vi "Dashboard Main.vi"() -> ()   [LabVIEW 2015]
uses:
  <vilib>/Utility/miscctls.llb/LVRowAndColumnTypeDef.ctl
  <vilib>/event_ctls.llb/eventvkey.ctl
  <vilib>/Rock Robotics/Network Tables/NT Write Boolean.vi
  <vilib>/Rock Robotics/WPI/Dashboard/WPI_DashboardLogging Global.vi
  <vilib>/Rock Robotics/Network Tables/NT Read Boolean.vi
  <vilib>/Utility/config.llb/Write Key (String).vi
  <vilib>/Utility/config.llb/Write Key (I32).vi
  <vilib>/Utility/config.llb/NI_LVConfig.lvlib
panel:
  out "camera num":string="Camera 1"
  out "Battery Voltage":bool
  out "timeLeft":dbl(slide) scale=0.0..150.0
  out "fps":dbl format="%#.1g"
  out "Mbps":dbl format="%#.1g"
  out "NT Connection":bool
  out "Mbps LED":bool
  in  "DB Camera Config":bool
  in  "TCP":refnum<k5>
  in  "Rec Mode":enum32{"Stop", "Record", "Playback"}(radio)
  in  "Vision":u16(ring) items=["Camera Off", "USB Camera SW", "USB Camera HW", "IP Camera"]
  out "Camera IP":string
  out "Image Message":string="Timeout in Camera Communications"
  in  "Dashboard Tab":T1(tab)
  out "Down":bool
  out "Up":bool
  out "readyToFire":bool
  out "aiming":bool
  in  "RPM setting":dbl=5400.0
  in  "Shot Mode":i32(listbox)
  in  "Defense":i32(listbox)
  in  "Autonomous Mode":i32(listbox)
  out "in range":bool
  out "back":bool
  out "forward":bool
  out "Distance":dbl
  out "Angle Off":dbl
  out "turn right":bool
  out "angleGood":bool
  out "turn left":bool
  in  "Camera Settings":T2={"Frame Rate"=30, "Compression"=30, "Size"=1} {"Frame Rate" scale=1.0..30.0; "Size" items=["640x480", "320x240", "160x120"]}
  out "Mode":T3(ring)=enum."Auto Disabled"
  out "processed image":T4(plugin-control)
  in  "rightSideSkew":dbl=0.2
  in  "leftSideSkew":dbl=1.8
  in  "compact max":dbl=1.0
  in  "compact min":dbl=0.2
  out "Shooter speed":dbl(knob) scale=0.0..6000.0
  in  "Test Slider":dbl(slide) scale=0.0..100.0 scale format="%#_3g"
  in  "On/Off":bool caption="Solenoid"
  in  "Test Name":u16(ring) items=["Select the test to run..."]
  in  "Test Tree":string(tree)
  in  "Motor":cluster{"Value":dbl, "Enable":bool} {"Value" scale=-1.0..1.0 scale format="%#_3g"}
  out "Progress":T5 {"Test Progress" scale=0.0..100.0}
  in  "Rev/Fwd":cluster{"Forward":bool, "Reverse":bool}
  in  "Test Ring":u16(ring) items=["Monochrome", "Color"]
  in  "hue max":dbl=115.0
  in  "sat max":dbl=255.0
  in  "val max":dbl=93.0
  in  "sat min":dbl=150.0
  in  "val min":dbl=9.0
  in  "hue min":dbl=90.0
  out "Cmd Status":string
  in  "Execute Command":bool
  in  "Command Params":string[][](table)
  in  "Command Selection":i32(listbox)
  in  "CheckList":i32(listbox)
  out "Tree":string(tree)
  out "Camera Image":T4(plugin-control)
  # "Range"
  # "Climber"
  # "Aim Direction"
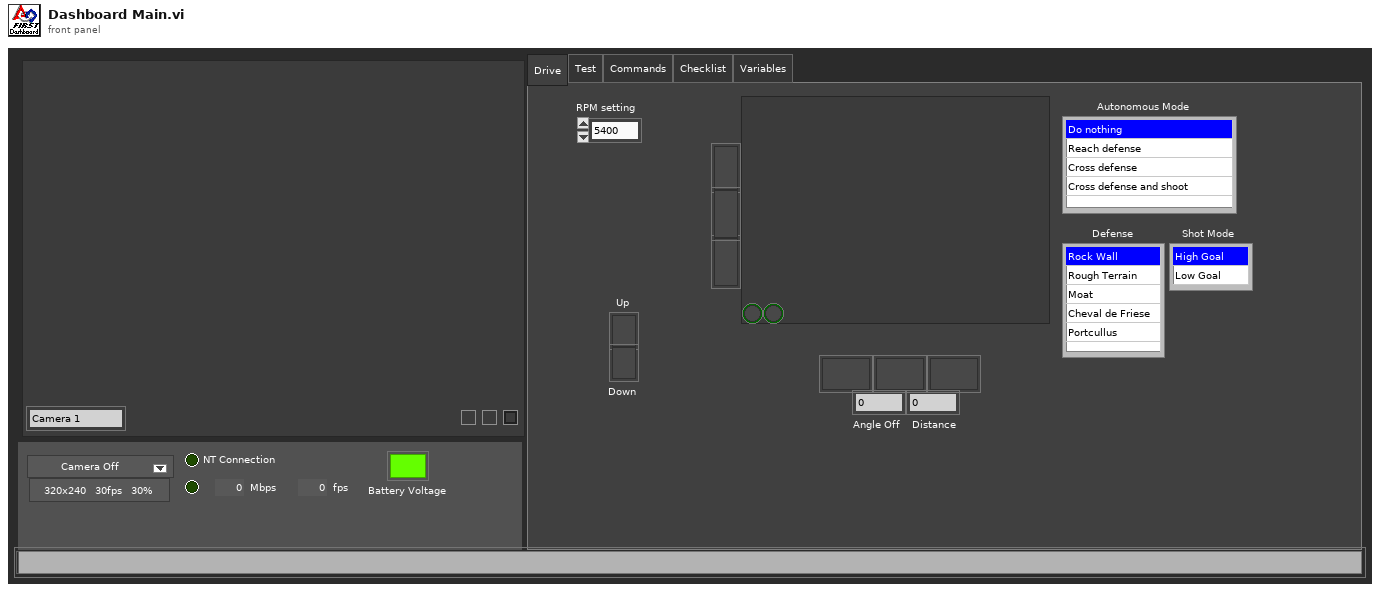
[diagram p1: front panel]
types:
  T1 = enum32{"Drive", "Test", "Commands", "Checklist", "Variables"}
  T2 = cluster{"Frame Rate":i32, "Compression":i32, "Size":u16}
  T3 = enum8{"Tele-Op Disabled", "Tele-Op Enabled", "Auto Disabled", "Auto Enabled", "Test Disabled", "Test Enabled", "Disconnected", "No Code", "E-Stop"}
  T4 = typedef "IMAQ Image.ctl" = refnum<image>
  T5 = cluster{"Test Progress":u8, "Test Progress Text":string}
  T6 = cluster{"IDs":cluster{"RPC field ID":u16, "Unique ID":u16}, "String":string}
  T7 = enum32{"Drive", "Basic", "Custom", "Test", "Checklist", "Variables"}
  T8 = typedef "Image Type" = u32
  T9 = cluster{"Error Strings":string, "Disable Counts":cluster{u16, u16}, "Rail Faults":cluster{u16, u16, u16}, "Robot IP":string, "DB Mode":u8, "Event Info":cluster{"Name":string, "Type":u8, "Number":u16, "Replay":u8}, "Camera Addr":string}
  T10 = cluster{"Storage":cluster{"Disk Free":u64, "RAM Block":u32, "RAM free":u32}, "CPU Utilization":cluster{"CPU % ISR":sgl, "CPU % Time Crit":sgl, "CPU % Timed Str":sgl, "CPU % High":sgl, "CPU % Above":sgl, "CPU % Normal":sgl, "CPU % Low":sgl}, "CAN":cluster{"% Bus Utilization":sgl, "Bus Off Cnt":u32, "TX_FIFO Full Cnt":u32, "Receive Error Cnt":u8, "Transmit Error Cnt":u8}, "HID":cluster{"HID Outputs":u32, "Rumble Low":u16, "Rumble High":u16}[]}
  T11 = cluster{"Status bits":cluster{"Test Mode":bool, "Autonomous":bool, "Enabled":bool, "Code Start":bool, "Brownout":bool, "Reserved 2":bool, "Reserved 3":bool, "E-Stop":bool}, "Code Trace":cluster{"Disabled":bool, "TeleOp":bool, "Auto":bool, "Test":bool}, "Controller Type":enum16{"unknown", "cRIO", "roboRio"}, "Code?":enum16{"unknown", "noCode", "code"}, "Battery V":dbl}
  T12 = cluster{"Control Bits":cluster{"TestMode":bool, "Autonomous":bool, "Enabled":bool, "FMS Present":bool, bool, bool, bool, "E-Stop":bool}, "Team Station ":u8, "Countdown":sgl, "Joystick Values":cluster{"Axes":dbl[], "Buttons":bool[], "POVs":i16[]}[]}
  T13 = cluster{cluster{"hue min":dbl, "hue max":dbl}, cluster{"sat min":dbl, "sat max":dbl}, cluster{"val min":dbl, "val max":dbl}}
  T14 = typedef "NI_LVConfig.lvlib/Config Data RefNum.ctl" = refnum<k1>
  T15 = cluster{"Operation":enum16{"Update", "Clear"}, "Color Box":u32}[]
  T16 = typedef "eventvkey.ctl" = enum16{"ASCII", "Enter", "Return", "Shift", "Ctrl", "Alt", "Cmd", "Opt", "Caps", "NumLock", "Clear", "Break", "Up", "Down", "Left", "Right", "Insert", "Delete", "Home", "End", "PageUp", "PageDown", "Escape", "Help", "Pause", "ScrollLock", "F1", "F2", "F3", "F4", "F5", "F6", "F7", "F8", "F9", "F10", "F11", "F12", "F13", "F14", "F15", "F16", "F17", "F18", "F19", "F20", "F21", "F22", "F23", "F24", "Play", "VolumeUp", "VolumeDown", "Mute", "Two Byte Char"}
  T17 = cluster{"Image Size":bool, "Image Type":bool, "Pixel Value":bool, "ROI Information":bool, "Zoom Factor":bool}
  T18 = enum8{"Enabled", "Disabled", "Disabled and Grayed Out"}
  T19 = cluster{"Operation":enum16{"Update", "Clear"}, "Color Box":u32}
  T20 = typedef "LVRowAndColumnTypeDef.ctl" = cluster{"Row":i32, "Column":i32}
  T21 = cluster{"Shift":bool, "Ctrl":bool, "Alt":bool, "Cmd":bool, "Opt":bool}
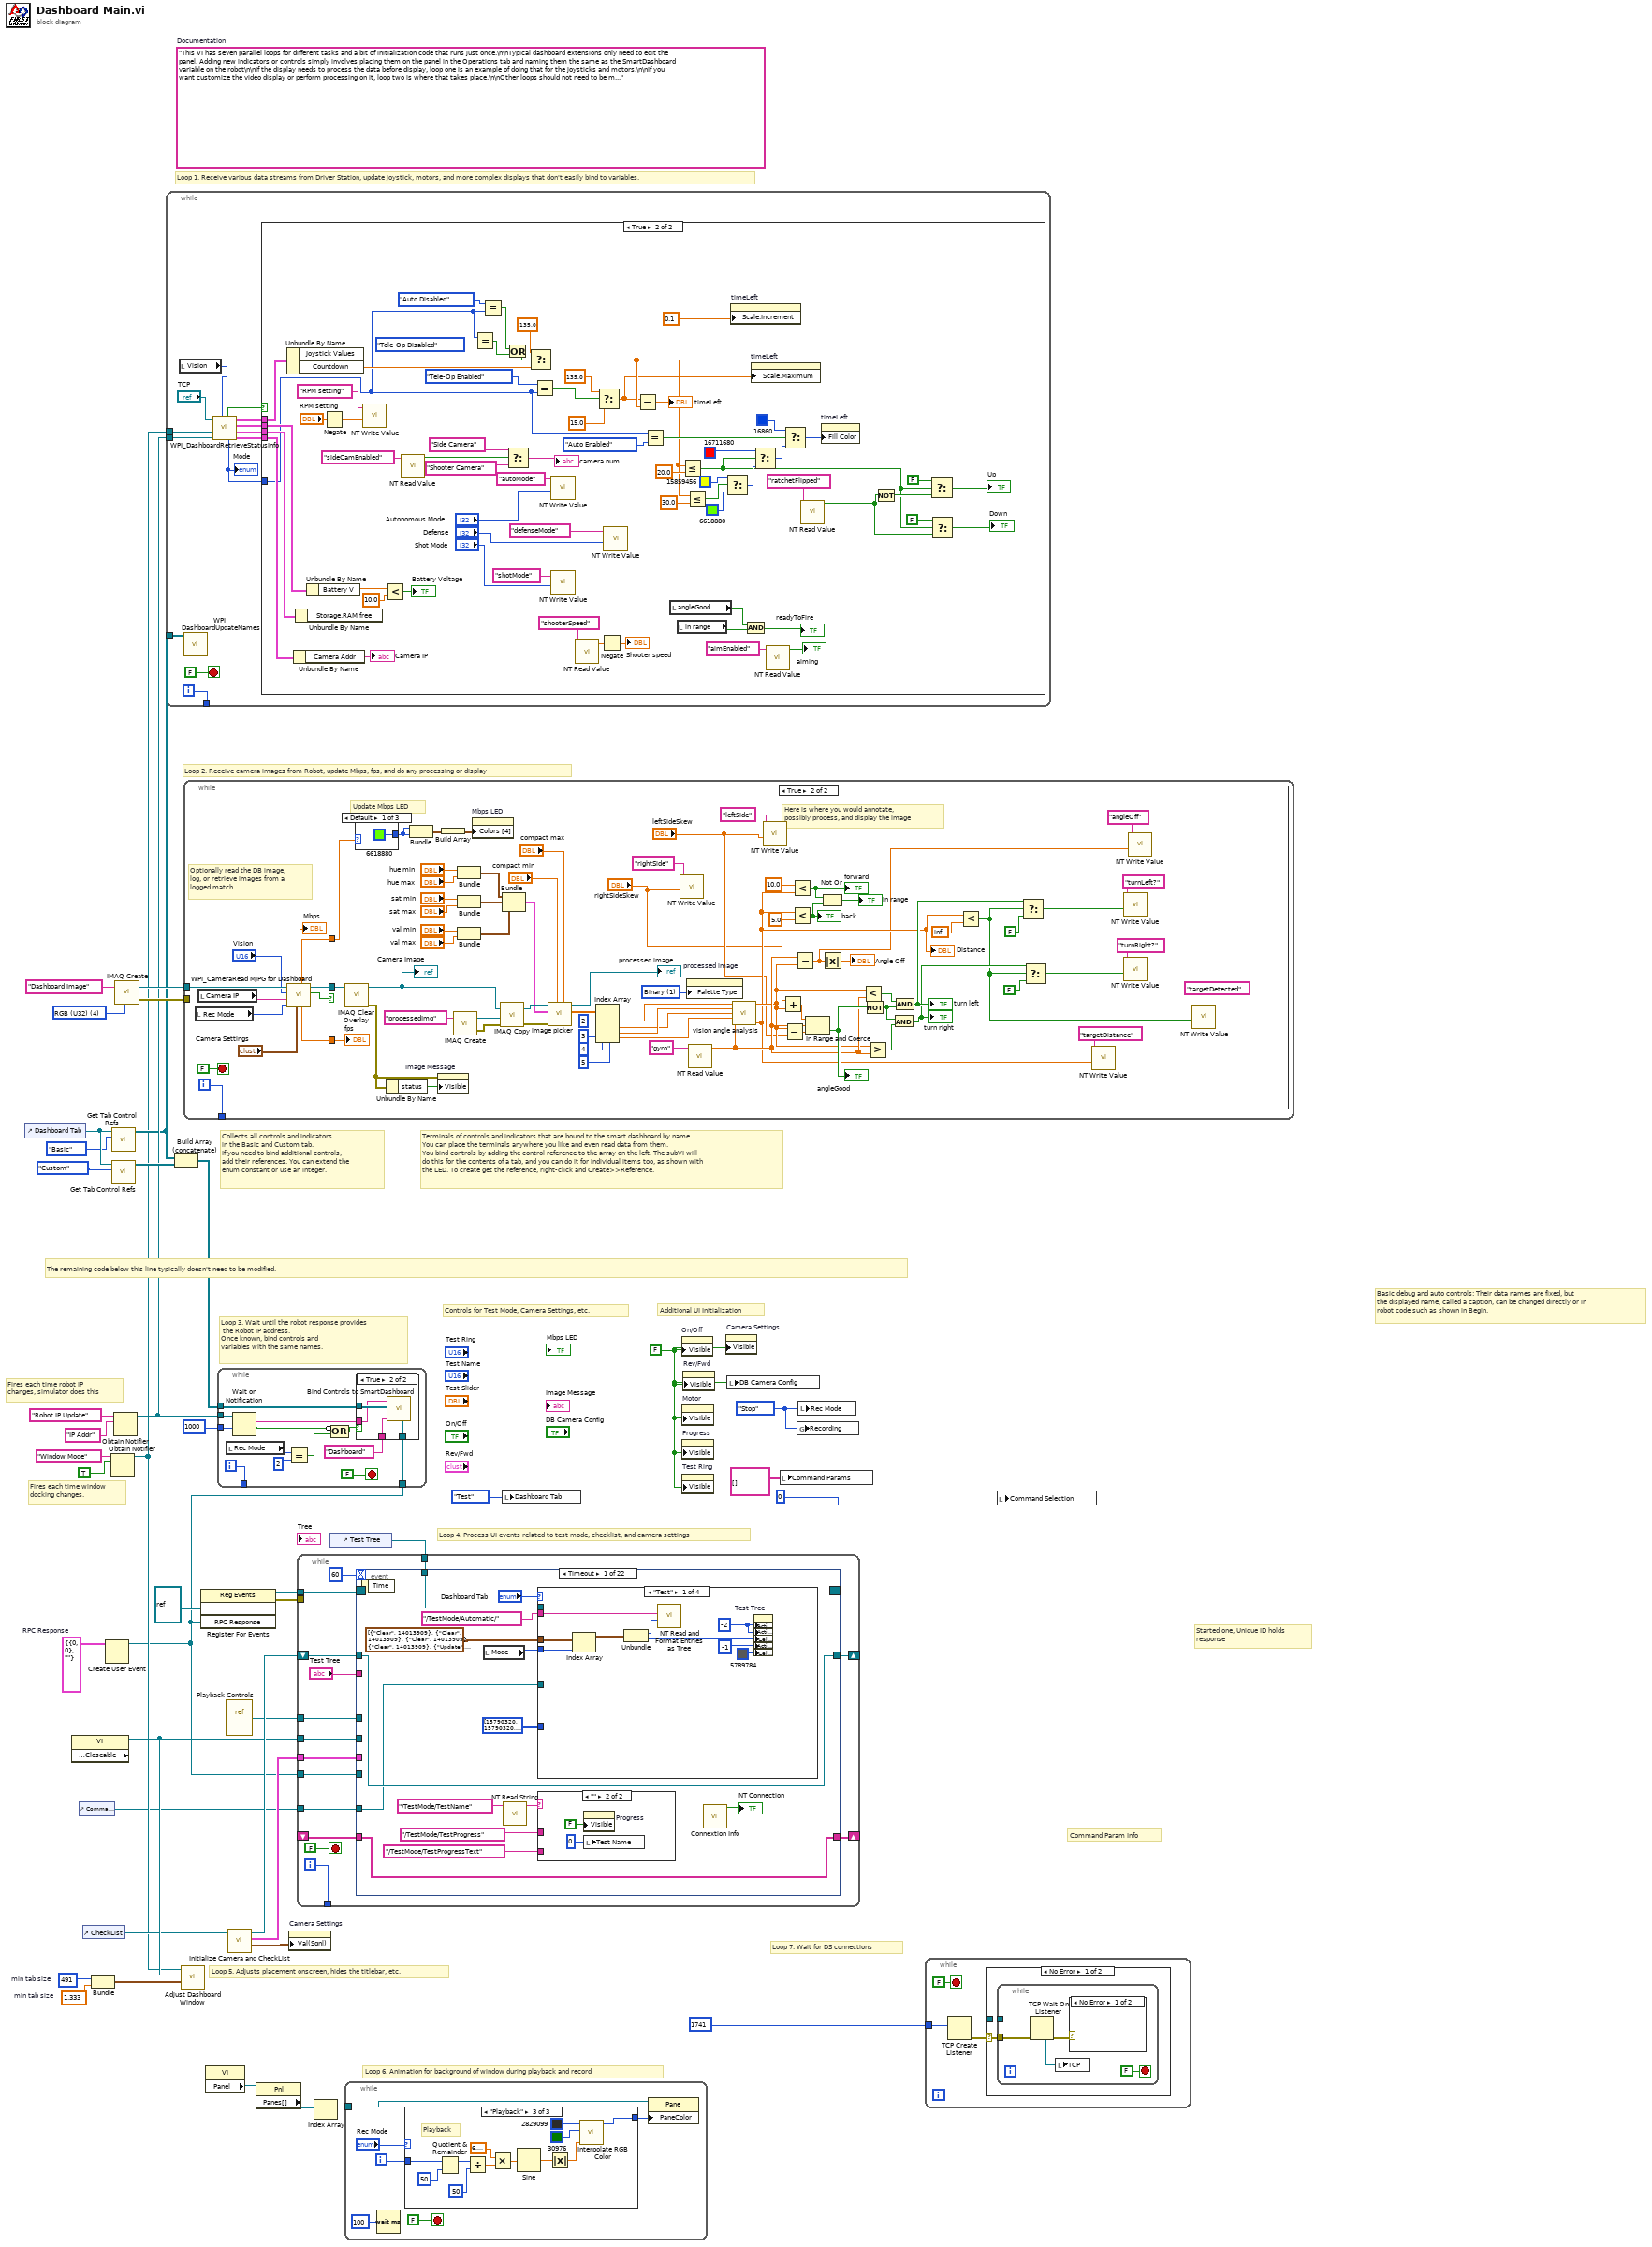
[diagram p0: block diagram]
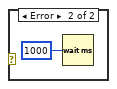
[diagram p2: hidden frame]
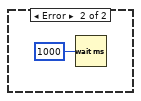
[diagram p3: hidden frame]
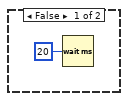
[diagram p4: hidden frame]
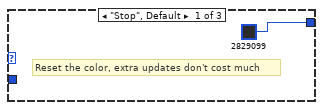
[diagram p5: hidden frame]
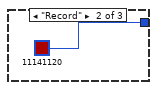
[diagram p6: hidden frame]
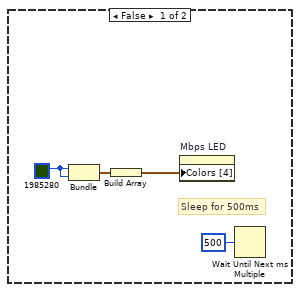
[diagram p8: hidden frame]
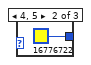
[diagram p9: hidden frame]
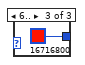
[diagram p10: hidden frame]
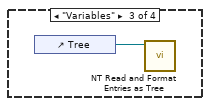
[diagram p12: hidden frame]
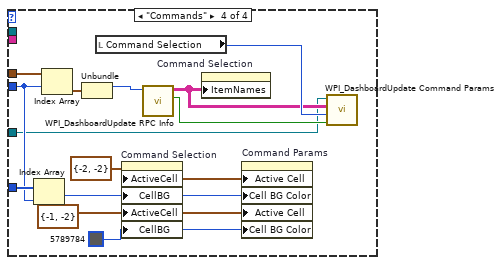
[diagram p13: hidden frame]
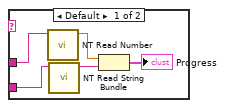
[diagram p14: hidden frame]
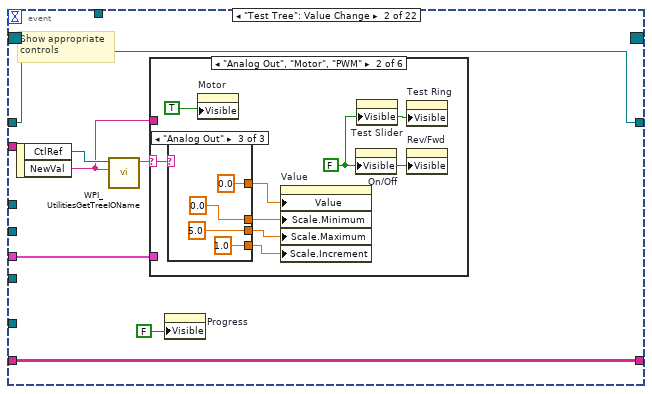
[diagram p15: hidden frame]
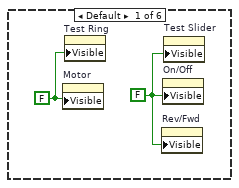
[diagram p16: hidden frame]
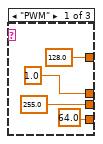
[diagram p17: hidden frame]
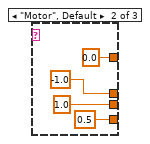
[diagram p18: hidden frame]
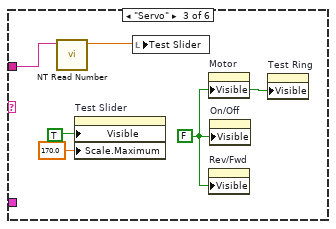
[diagram p19: hidden frame]
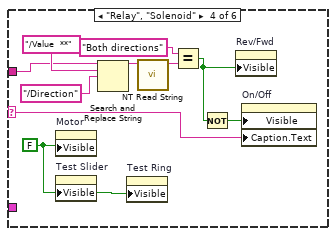
[diagram p20: hidden frame]
diagram:
  w5 = T6 {"IDs"={"RPC field ID"=0, "Unique ID"=0}, "String"=""}  # RPC Response
  w17 = 491  # min tab size
  w16 = 1.333  # min tab size
  w22 = enum32{"Stop", "Record", "Playback"}."Stop" ("Rec Mode")
  w11 = FALSE ("Visible")
  (unwired) "This VI has seven parallel loops for different tasks and a bit of initialization code that runs just once.\n\nTypical dashboard extensions only need to edit the panel. Adding new indicators or controls simply involves placing them on the panel in the Operations tab and naming them the same as the SmartDashboard variable on the robot\n\nIf the display needs to process the data before display, loop one is an example of doing that for the joysticks and motors.\n\nIf you want customize the video display or perform processing on it, loop two is where that takes place.\n\nOther loops should not need to be modified. They are pretty standard, and document the task they perform."  # Documentation
  w42 = T8 4 items=["Grayscale (U8)", "Grayscale (I16)", "Grayscale (SGL)", "Complex (CSG)", "RGB (U32)", "HSL (U32)", "RGB (U64)"] ("Image Type")
  # "Command Param Info"
  # "Started one, Unique ID holds\nresponse"
  # "Loop 7. Wait for DS connections"
  # "Basic debug and auto controls: Their data names are fixed, but\nthe displayed name, called a caption, can be changed directly or in\nrobot code such as shown in Begin."
  # "Controls for Test Mode, Camera Settings, etc."
  # "Additional UI Initialization"
  # "Loop 6. Animation for background of window during playback and record"
  # "Fires each time robot IP\nchanges, simulator does this"
  # "Fires each time window\ndocking changes."
  # "Collects all controls and indicators\nin the Basic and Custom tab.\nIf you need to bind additional controls,\nadd their references. You can extend the\nenum constant or use an integer."
  # "The remaining code below this line typically doesn't need to be modified."
  # "Loop 4. Process UI events related to test mode, checklist, and camera settings"
  # "Terminals of controls and indicators that are bound to the smart dashboard by name.\nYou can place the terminals anywhere you like and even read data from them.\nYou bind controls by adding the control reference to the array on the left. The subVI will\ndo this for the contents of a tab, and you can do it for individual items too, as shown with\nthe LED. To create get the reference, right-click and Create>>Reference."
  # "Loop 3. Wait until the robot response provides\n the Robot IP address.\nOnce known, bind controls and\nvariables with the same names."
  # "Loop 5. Adjusts placement onscreen, hides the titlebar, etc."
  # "Loop 1. Receive various data streams from Driver Station, update joystick, motors, and more complex displays that don't easily bind to variables."
  # "Loop 2. Receive camera images from Robot, update Mbps, fps, and do any processing or display"
  n1 = control-ref of="Dashboard Tab"() -> (w20:refnum<vi>)
  n2 = property class="VI" props=["Front Panel.Closeable"]() -> (reference out=w21:refnum<vi>)  [unwired: 2 in, 2 out]
  n3 = control-ref of="Command Params"() -> (w1:refnum<vi>)
  n4 = control-ref of="CheckList"() -> (w12:refnum<vi>)
  n5 = Bundle("min tab size"=w17, "min tab size"=w16) -> (w15:cluster{"min tab size":i32, "min tab size":dbl})  [unwired: 1 in]
  n6 = Create User Event(user event datatype=w5) -> (user event=w2:refnum<user-event>)  [unwired: 1 in, 1 out]
  n7 = Obtain Notifier(name (unnamed)="Window Mode", notification data type=TRUE) -> (notifier out=w8:refnum<notifier>)  [unwired: 2 in, 2 out]
  n8 = call <vilib>:"Get Tab Control Refs.vi"("Page Index"=T7."Basic" ("Dashboard Tab"), "TabControl in"=w20) -> ("ControlsOnPage"=w9:refnum<vi>[])  [unwired: 9 in]
  n9 = call <vilib>:"Get Tab Control Refs.vi"("Page Index"=T7."Custom" ("Dashboard Tab"), "TabControl in"=w20) -> ("ControlsOnPage"=w19:refnum<vi>[])  [unwired: 9 in]
  n10 = Obtain Notifier(name (unnamed)="Robot IP Update", notification data type="IP Addr" ("name (unnamed)")) -> (notifier out=w10:refnum<notifier>)  [unwired: 2 in, 2 out]
  n11 = call "IMAQ Create"("Image Name"="Dashboard Image", "Image Type"=w42) -> ("New Image"=w40:T4, "error out"=w39:errorcluster)  [unwired: 2 in, 1 out]
  n12 = while {
    tunnel: [w54] -> _
    tunnel: w10 -> [w48]
    tunnel: w9 -> [w47]
    tunnel: w8 -> [w43]
    i -> [w54]
    stop <- FALSE stop-if-true
    n13 = local read "Vision"() -> (w45:u16)
    n14 = call <vilib>:"WPI_DashboardUpdateNames.vi"("Controls on Tab"=w47) -> ()  [unwired: 11 in]
    n15 = call <vilib>:"WPI_DashboardRetrieveStatusInfo.vi"("Vision"=w45, "Binding Refnum"=w48, "Window Mode Notifier"=w43, "TCP Cnx"="TCP") -> ("Power and Errors"=w49:T9, "Robot Metrics"=w52:T10, "Status Info"=w53:T11, "Control Info"=w50:T12, "Robot Mode"=w46:T3, "Process?"=w51:bool)  [unwired: 2 in]
    "Mode" <- w46
    n16 = case shown="True" w51 {
      tunnel: w53 -> [_ w122]
      tunnel: w52 -> [_ w121]
      tunnel: w50 -> [_ w120]
      tunnel: w49 -> [_ w119]
      tunnel: w46 -> [_ w67]
      frame False {
        n17 = Wait (ms)(milliseconds to wait=u32 20) -> ()  [unwired: 1 out]
      }
      frame True {
        n18 = Unbundle By Name(w120) -> ("Countdown"=w82:sgl)  [unwired: 1 out]
        n19 = Unbundle By Name(w119) -> ("Camera Addr"=→"Camera IP":string)
        n20 = Unbundle By Name(w121) -> ()  [unwired: 1 out]
        n21 = Unbundle By Name(w122) -> ("Battery V"=w117:dbl)
        n22 = Negate(x="RPM setting") -> (-x=w94:dbl)
        n23 = call-poly <vilib>:"NT Write Value.vi"("Numeric"=w94, "Name"="RPM setting") -> ()  [unwired: 9 in, 1 out]
        n24 = Less?(x=w117, y=10.0) -> (x < y?=→"Battery Voltage":bool)
        n25 = call-poly <vilib>:"NT Read Value.vi"("Name"="sideCamEnabled") -> ("Boolean"=w111:bool)  [unwired: 9 in, 1 out]
        n26 = Equal?(x=w67, y=T3."Tele-Op Disabled") -> (x = y?=w68:bool)
        n27 = Equal?(x=T3."Auto Disabled" ("Robot Mode"), y=w67) -> (x = y?=w69:bool)
        n28 = Or(x=w69, y=w68) -> (x .or. y?=w70:bool)
        n29 = Select(t="Side Camera", s=w111, f="Shooter Camera") -> (s? t:f=→"camera num":string)
        n30 = Select(t=sgl 135.0, s=w70, f=w82) -> (s? t:f=w74:sgl)
        n31 = Equal?(x=T3."Tele-Op Enabled" ("Robot Mode"), y=w67) -> (x = y?=w76:bool)
        n32 = call-poly <vilib>:"NT Write Value.vi"("Numeric"="Autonomous Mode", "Name"="autoMode") -> ()  [unwired: 9 in, 1 out]
        n33 = call-poly <vilib>:"NT Write Value.vi"("Numeric"="Shot Mode", "Name"="shotMode") -> ()  [unwired: 9 in, 1 out]
        n34 = call-poly <vilib>:"NT Read Value.vi"("Name"="shooterSpeed") -> ("Numeric"=w105:dbl)  [unwired: 9 in, 1 out]
        n35 = Select(t=135.0, s=w76, f=15.0) -> (s? t:f=w72:dbl)
        n36 = Negate(x=w105) -> (-x=→"Shooter speed":dbl)
        n37 = call-poly <vilib>:"NT Write Value.vi"("Numeric"="Defense", "Name"="defenseMode") -> ()  [unwired: 9 in, 1 out]
        n38 = Subtract(x=w72, y=w74) -> (x-y=→"timeLeft":dbl)
        n39 = Equal?(x=w67, y=T3."Auto Enabled") -> (x = y?=w88:bool)
        n40 = local read "angleGood"() -> (w95:bool)
        n41 = local read "in range"() -> (w96:bool)
        n42 = Less Or Equal?(x=w74, y=sgl 20.0) -> (x <= y?=w59:bool)
        n43 = Less Or Equal?(x=w74, y=sgl 30.0) -> (x <= y?=w79:bool)
        n44 = Select(t=u32 15859456, s=w79, f=u32 6618880) -> (s? t:f=w80:u32)
        n45 = property on="timeLeft" class="Slide (strict)"("Scale.Increment"=0.1 ("Scale.Range:Increment")) -> ()  [unwired: 2 in, 2 out]
        n46 = And(x=w95, y=w96) -> (x .and. y?=→"readyToFire":bool)
        n47 = property on="timeLeft" class="Slide (strict)"("Scale.Maximum"=w72) -> ()  [unwired: 2 in, 2 out]
        n48 = Select(t=u32 16711680, s=w59, f=w80) -> (s? t:f=w83:u32)
        n49 = call-poly <vilib>:"NT Read Value.vi"("Name"="aimEnabled") -> ("Boolean"=→"aiming":bool)  [unwired: 9 in, 1 out]
        n50 = Select(t=u32 16860, s=w88, f=w83) -> (s? t:f=w86:u32)
        n51 = call-poly <vilib>:"NT Read Value.vi"("Name"="ratchetFlipped") -> ("Boolean"=w60:bool)  [unwired: 9 in, 1 out]
        n52 = property on="timeLeft" class="Slide (strict)"("Fill Color"=w86) -> ()  [unwired: 2 in, 2 out]
        n53 = Not(x=w60) -> (.not. x?=w61:bool)
        n54 = Select(t=FALSE, s=w59, f=w61) -> (s? t:f=→"Up":bool)
        n55 = Select(t=FALSE, s=w59, f=w60) -> (s? t:f=→"Down":bool)
      }
    }
  }
  n56 = Build Array (concatenate)(w9, w19) -> (w18:refnum<vi>[])
  n57 = call "Adjust Dashboard Window.vi"("Size Constraints"=w15, "VI"=w21, "WIn Mode"=w8) -> ()  [unwired: 9 in]
  n58 = while {
    tunnel: w40 -> [w131]
    tunnel: w39 -> [_]
    tunnel: [w132] -> _
    i -> [w132]
    stop <- FALSE stop-if-true
    # "Optionally read the DB image,\nlog, or retrieve images from a\nlogged match"
    n59 = local read "Rec Mode"() -> (w126:enum32{"Stop", "Record", "Playback"})
    n60 = local read "Camera IP"() -> (w124:string)
    n61 = call <vilib>:"WPI_CameraRead MJPG for Dashboard.vi"("Camera Settings"="Camera Settings", "Rec Mode"=w126, "Camera IP"=w124, "Camera Mode"="Vision", "Refnum in"=w131) -> ("Active"=w129:bool, "Refnum out"=w130:T4, "FPS"=w128:dbl, "Bandwidth (Mbps)"=w123:dbl)  [unwired: 3 in]
    "Mbps" <- w123
    n62 = case shown="True" w129 {
      tunnel: w130 -> [_ w204]
      tunnel: w123 -> [_ w203]
      tunnel: w128 -> [_ w202]
      frame False {
        w134 = u32 1985280 ("Color Box")
        # "Sleep for 500ms"
        n63 = Bundle("Color Box"=w134, "Color Box"=w134) -> (w136:cluster{"Color Box":u32, "Color Box":u32})  [unwired: 1 out]
        n64 = Build Array(w136) -> (w135:cluster{"Color Box":u32, "Color Box":u32}[])
        n65 = property on="Mbps LED" class="Bool (strict)"("Colors [4]"=w135) -> ()  [unwired: 2 in, 2 out]
        n66 = Wait Until Next ms Multiple(millisecond multiple=u32 500) -> ()  [unwired: 1 out]
      }
      frame True {
        w178 = u32 1 items=["Grayscale", "Binary", "Gradient", "Rainbow", "Temperature", "User Defined", "Binary 16 Bit", "Gradient 16 Bit", "Rainbow 16 Bit", "Temperature 16 Bit", "User Defined 16 Bit"] ("Palette:Palette Type")
        # "Here is where you would annotate,\npossibly process, and display the image"
        # "Update Mbps LED"
        n67 = call "IMAQ Clear Overlay"("Image"=w204) -> ("error out"=w201:errorcluster, "Image Out"=w182:T4)  [unwired: 2 in, 7 out]
        "Camera Image" <- w182
        n68 = case shown="Default" w203 {
          tunnel: [u32 6618880 ("Color Box") u32 16776722 ("Color Box") u32 16716800 ("Color Box")] -> w205
          frame Default {
          }
          frame 4, 5 {
          }
          frame 6.. {
          }
        }
        n69 = Unbundle By Name(w201) -> ("status"=w208:bool)
        n70 = Bundle("Color Box"=w205, "Color Box"=w205) -> (w207:cluster{"Color Box":u32, "Color Box":u32})  [unwired: 1 out]
        n71 = property on="Image Message" class="Str"(error in=w201, "Visible"=w208) -> ()  [unwired: 1 in, 2 out]
        n72 = Build Array(w207) -> (w206:cluster{"Color Box":u32, "Color Box":u32}[])
        n73 = call "IMAQ Create"("Image Name"="processedImg") -> ("New Image"=w181:T4, "error out"=w180:errorcluster)  [unwired: 4 in]
        n74 = Bundle("hue min"="hue min", "hue max"="hue max") -> (w175:cluster{"hue min":dbl, "hue max":dbl})  [unwired: 1 in]
        n75 = Bundle("sat min"="sat min", "sat max"="sat max") -> (w176:cluster{"sat min":dbl, "sat max":dbl})  [unwired: 1 in]
        n76 = Bundle("val min"="val min", "val max"="val max") -> (w177:cluster{"val min":dbl, "val max":dbl})  [unwired: 1 in]
        n77 = property on="Mbps LED" class="Bool (strict)"("Colors [4]"=w206) -> ()  [unwired: 2 in, 2 out]
        n78 = call "IMAQ Copy"("error in (no error)"=w180, "Image Dst"=w181, "Image Src"=w182) -> ("error out"=w184:errorcluster, "Image Dst Out"=w183:T4)  [unwired: 3 in]
        n79 = Bundle(w175, w176, w177) -> (w169:T13)  [unwired: 1 in]
        n80 = call "image picker.vi"("compactnessMax"="compact max", "compactnessMin"="compact min", "error in"=w184, "rgb constants"=w169, "Image In"=w183) -> ("report"=w167:dbl[], "Image Out"=→"processed image":T4)  [unwired: 4 in, 1 out]
        n81 = Index Array(array=w167, index #1=2 ("index"), index #2=3 ("index"), index #3=4 ("index"), index #4=5 ("index")) -> (element #1=w162:dbl, element #2=w160:dbl, element #3=w161:dbl, element #4=w159:dbl)
        n82 = call-poly <vilib>:"NT Write Value.vi"("Numeric"="rightSideSkew", "Name"="rightSide") -> ()  [unwired: 9 in, 1 out]
        n83 = property on="processed image" class="ImageControl"("Palette Type"=w178) -> ()  [unwired: 2 in, 2 out]
        n84 = call-poly <vilib>:"NT Read Value.vi"("Name"="gyro") -> ("Numeric"=w192:dbl)  [unwired: 9 in, 1 out]
        n85 = call "vision angle analysis.vi"("left_x"=w162, "right_x"=w161, "top_y"=w160, "bottom_y"=w159, "gyro_angle_deg"=w192) -> ("gyro_heading_deg"=w154:dbl, "distance"=w147:dbl)  [unwired: 9 in]
        "Distance" <- w147
        n86 = call-poly <vilib>:"NT Write Value.vi"("Numeric"="leftSideSkew", "Name"="leftSide") -> ()  [unwired: 9 in, 1 out]
        n87 = Add(x="rightSideSkew", y=w154) -> (x+y=w197:dbl)
        n88 = Subtract(x=w154, y="leftSideSkew") -> (x-y=w198:dbl)
        n89 = Less?(x=10.0, y=w147) -> (x < y?=w189:bool)
        "forward" <- w189
        n90 = Less?(x=w147, y=5.0) -> (x < y?=w188:bool)
        "back" <- w188
        n91 = Subtract(x=w192, y=w154) -> (x-y=w143:dbl)
        n92 = In Range and Coerce(upper limit=w197, x=w192, lower limit=w198) -> (In Range?=w196:bool)  [unwired: 1 out]
        "angleGood" <- w196
        n93 = Not Or(1:w188, 2:w189) -> (0:→"in range":bool)
        n94 = Absolute Value(x=w143) -> (abs(x)=→"Angle Off":dbl)
        n95 = Less?(x=w154, y=w192) -> (x < y?=w193:bool)
        n96 = Not(x=w196) -> (.not. x?=w195:bool)
        n97 = Greater?(x=w154, y=w192) -> (0:w194:bool)
        n98 = And(x=w195, y=w194) -> (x .and. y?=w150:bool)
        "turn right" <- w150
        n99 = And(x=w193, y=w195) -> (x .and. y?=w153:bool)
        "turn left" <- w153
        n100 = Less?(x=w147, y=inf) -> (x < y?=w144:bool)
        n101 = Select(t=w153, s=w144, f=FALSE) -> (s? t:f=w152:bool)
        n102 = Select(t=w150, s=w144, f=FALSE) -> (s? t:f=w148:bool)
        n103 = call-poly <vilib>:"NT Write Value.vi"("Numeric"=w147, "Name"="targetDistance") -> ()  [unwired: 9 in, 1 out]
        n104 = call-poly <vilib>:"NT Write Value.vi"("Boolean"=w152, "Name"="turnLeft?") -> ()  [unwired: 9 in, 1 out]
        n105 = call-poly <vilib>:"NT Write Value.vi"("Boolean"=w148, "Name"="turnRight?") -> ()  [unwired: 9 in, 1 out]
        n106 = call-poly <vilib>:"NT Write Value.vi"("Numeric"=w143, "Name"="angleOff") -> ()  [unwired: 9 in, 1 out]
        n107 = call-poly <vilib>:"NT Write Value.vi"("Boolean"=w144, "Name"="targetDetected") -> ()  [unwired: 9 in, 1 out]
        "fps" <- w202
      }
    }
  }
  n108 = register-events(refnum<vi> refnum, w2) -> (reference out=w26:refnum<event-registration>, error out=w25:errorcluster)  [unwired: 2 in]
  n109 = property class="VI"() -> ("Panel"=w29:refnum<vi>)  [unwired: 2 in, 2 out]
  n110 = while {
    tunnel: w18 -> [w224]
    tunnel: w10 -> [w222]
    tunnel: [w220] -> _
    tunnel: u32 1000 ("milliseconds to wait") -> [w219]
    tunnel: w2 -> [w212]
    i -> [w220]
    stop <- FALSE stop-if-true
    n111 = local read "Rec Mode"() -> (w215:enum32{"Stop", "Record", "Playback"})
    n112 = Wait on Notification(notifier=w222, timeout in ms (-1)=w219) -> (notification=w221:string, timed out?=w217:bool)  [unwired: 2 in, 2 out]
    n113 = Equal?(x=w215, y=u16 2 ("Rec Mode")) -> (x = y?=w216:bool)
    n114 = Compound Arithmetic op=OR(invert w217, w216) -> (w218:bool)
    n115 = case shown="True" w218 {
      tunnel: w224 -> [_ w228]
      tunnel: w221 -> [_ w227]
      tunnel: "Dashboard" -> [_ w226]
      tunnel: w212 -> [_ w225]
      frame False {
      }
      frame True {
        n116 = call <vilib>:"Bind Controls to SmartDashboard.vi"("RPC ref"=w225, "Client Name"=w226, "Bound Control Refs"=w228, "Server IP Address"=w227) -> ()  [unwired: 8 in]
      }
    }
  }
  n117 = vi-ref "Playback Controls.vi"() -> (w27:refnum<vi>)
  n118 = call "Initialize Camera and CheckList.vi"("ListBox in"=w12) -> ("Cluster"=w33:cluster{"value":i32, "value":i32, "index":i32}, "Array"=w34:cluster{string[]}[], "File Refnum"=w32:T14)  [unwired: 8 in]
  n119 = property class="Pnl"(reference=w29) -> ("Panes[]"=w30:refnum<vi>[])  [unwired: 1 in, 2 out]
  n120 = property on="Camera Settings" class="Clust (strict)"("Val(Sgnl)"=w33) -> ()  [unwired: 2 in, 2 out]
  n121 = Index Array(array=w30) -> (element=w28:refnum<vi>)  [unwired: 1 in]
  n122 = control-ref of="Test Tree"() -> (w31:refnum<vi>)
  n123 = while {
    tunnel: w34 -> [w240]
    shift-right: [w239] -> _
    shift-left: w32 -> [w238]
    tunnel: [w237] -> _
    tunnel: w31 -> [w236]
    tunnel: w27 -> [w235]
    tunnel: w26 -> [w234]
    tunnel: w25 -> [_]
    tunnel: w21 -> [w233]
    tunnel: w2 -> [w232]
    tunnel: w1 -> [w231]
    shift-right: [w230] -> _
    shift-left: _ -> [w229]
    i -> [w237]
    stop <- FALSE stop-if-true
    n124 = event shown="[0] Timeout" {
      selector: w234 -> [_ _ _ _ _ _ _ _ _ _ _ _ _ _ _ _ _ _ _ _ _ _]
      dyn-events: [_ _ _ _ _ _ _ _ _ _ _ _ _ _ _ _ w541 _ _ _ _ _] -> _
      timeout: u32 60 ("milliseconds to wait") -> [_ _ _ _ _ _ _ _ _ _ _ _ _ _ _ _ _ _ _ _ _ _]
      tunnel: w236 -> [w253 _ _ _ _ _ _ _ _ _ _ _ _ _ _ _ _ _ _ _ _ _]
      tunnel: "Test Tree" -> [_ _ _ _ _ _ _ _ _ _ _ w504 w513 w516 w521 w530 _ _ _ _ _ _]
      tunnel: w240 -> [_ w291 _ _ _ _ _ _ _ w466 w497 _ _ _ _ _ _ _ _ _ _ _]
      tunnel: [w250 w290 w394 w400 w412 w424 w432 w438 w451 w465 w490 w503 w511 w515 w520 w529 w543 w559 w561 w569 w580 w585] -> w239
      tunnel: w238 -> [w250 w290 w394 w400 w412 w424 w432 w438 w451 w464 w490 w503 w511 w515 w520 w529 w543 w559 w561 w569 w580 w585]
      tunnel: w235 -> [_ _ _ _ _ _ _ _ _ _ _ _ _ _ _ _ w544 _ w564 _ _ _]
      tunnel: w233 -> [_ _ _ _ _ _ _ _ _ _ _ _ _ _ _ _ w539 _ _ _ _ _]
      tunnel: w232 -> [_ _ _ _ _ _ _ _ _ _ _ _ _ _ _ _ w535 _ _ _ _ _]
      tunnel: w231 -> [w245 _ _ _ w410 _ _ _ _ _ _ _ _ _ _ _ _ _ _ _ _ _]
      tunnel: [w244 w289 w393 w399 w408 w418 w429 w437 w450 w463 w489 w502 w510 w514 w519 w528 w534 w557 w560 w565 w573 w586] -> w230
      tunnel: w229 -> [w244 w289 w393 w399 w408 _ _ w437 w450 w463 w489 w502 w510 w514 w519 w528 w534 w557 w560 w565 w573 w586]
      event Timeout {
        n125 = event-data() -> ()  [unwired: 1 in, 1 out]
        n126 = local read "Mode"() -> (w247:T3)
        n127 = call <vilib>:"NT Read String.vi"("Name"="/TestMode/TestName") -> ("String"=w256:string)  [unwired: 9 in, 1 out]
        n128 = case shown="\"Test\"" "Dashboard Tab" {
          tunnel: w253 -> [w267 _ _ _]
          tunnel: "/TestMode/Automatic/" ("Name Pattern") -> [w266 _ _ _]
          tunnel: T15 [{"Operation"=enum."Clear", "Color Box"=14013909}, {"Operation"=enum."Clear", "Color Box"=14013909}, {"Operation"=enum."Clear", "Color Box"=14013909}, {"Operation"=enum."Clear", "Color Box"=14013909}, {"Operation"=enum."Update", "Color Box"=14013909}, {"Operation"=enum."Update", "Color Box"=16777215}, {"Operation"=enum."Clear", "Color Box"=14013909}, {"Operation"=enum."Clear", "Color Box"=14013909}, {"Operation"=enum."Clear", "Color Box"=14013909}] -> [w259 _ _ w276]
          tunnel: w247 -> [w258 _ _ w275]
          tunnel: u32[] [15790320, 15790320, 15790320, 15790320, 16777215, 16777215, 15790320, 15790320, 15790320] -> [_ _ _ w281]
          tunnel: w245 -> [_ _ _ w269]
          frame "Test" {
            w265 = -2 ("Active Item:Row Number")
            n129 = Index Array(array=w259, index=w258) -> (element=w260:T19)
            n130 = Unbundle(w260) -> ("Operation"=w261:enum16{"Update", "Clear"}, "Color Box"=w262:u32)
            n131 = call <vilib>:"NT Read and Format Entries as Tree.vi"("Operation"=w261, "Name Pattern"=w266, "Tree Refnum"=w267) -> ()  [unwired: 7 in, 2 out]
            n132 = property on="Test Tree" class="Tree (strict)"("Active Item Row Number"=w265, "ActiveColNum"=w265, "CellBG"=w262, "Active Item Row Number"=-1 ("Active Item:Row Number"), "CellBG"=u32 5789784 ("Color Box")) -> ()  [unwired: 2 in, 2 out]
          }
          frame Default {
          }
          frame "Variables" {
            n133 = control-ref of="Tree"() -> (w268:refnum<vi>)
            n134 = call <vilib>:"NT Read and Format Entries as Tree.vi"("Tree Refnum"=w268) -> ()  [unwired: 9 in, 2 out]
          }
          frame "Commands" {
            w277 = u32 5789784 ("Color Box")
            w278 = T20 {"Row"=-1, "Column"=-2} ("Active Cell:Active Cell")
            w280 = T20 {"Row"=-2, "Column"=-2} ("Active Cell:Active Cell")
            n135 = Index Array(array=w281, index=w275) -> (element=w279:u32)
            n136 = Index Array(array=w276, index=w275) -> (element=w274:T19)
            n137 = Unbundle(w274) -> ("Operation"=w273:enum16{"Update", "Clear"})  [unwired: 1 out]
            n138 = local read "Command Selection"() -> (w272:i32)
            n139 = property on="Command Selection" class="MCListbox (strict)"("ActiveCell"=w280, "CellBG"=w279, "ActiveCell"=w278, "CellBG"=w277) -> ()  [unwired: 2 in, 2 out]
            n140 = call <vilib>:"WPI_DashboardUpdate RPC Info.vi"("Operation"=w273) -> ("update"=w271:bool, "commands"=w270:string[][])  [unwired: 9 in]
            n141 = property on="Command Selection" class="MCListbox (strict)"("ItemNames"=w270) -> ()  [unwired: 2 in, 2 out]
            n142 = property on="Command Params" class="Tbl (strict)"("Active Cell"=w280, "Cell BG Color"=w279, "Active Cell"=w278, "Cell BG Color"=w277) -> ()  [unwired: 2 in, 2 out]
            n143 = call <vilib>:"WPI_DashboardUpdate Command Params.vi"("Update"=w271, "NewVal"=w272, "Commands"=w270, "Param Tbl"=w269) -> ()  [unwired: 7 in, 1 out]
          }
        }
        n144 = case shown="\"\"" w256 {
          tunnel: "/TestMode/TestProgress" ("Name") -> [w283 _]
          tunnel: "/TestMode/TestProgressText" ("Name") -> [w282 _]
          frame Default {
            n145 = call <vilib>:"NT Read Number.vi"("Name"=w283) -> ("Numeric"=w284:dbl)  [unwired: 9 in, 1 out]
            n146 = call <vilib>:"NT Read String.vi"("Name"=w282) -> ("String"=w285:string)  [unwired: 9 in, 1 out]
            n147 = Bundle("Numeric"=w284, "String"=w285) -> (→"Progress":cluster{"Numeric":dbl, "String":string})  [unwired: 1 in]
          }
          frame "" {
            n148 = property on="Progress" class="Clust (strict)"("Visible"=FALSE) -> ()  [unwired: 2 in, 2 out]
            n149 = local write "Test Name"(u16 0) -> ()
          }
        }
        n150 = call <vilib>:"Connextion Info.vi"() -> ("Connected"=→"NT Connection":bool)  [unwired: 10 in, 1 out]
      }
      event "Test Tree": Value Change {
        # "Show appropriate\ncontrols"
        n151 = event-data() -> ("CtlRef"=w294:refnum<vi>, "NewVal"=w292:string)  [unwired: 1 in]
        n152 = call <vilib>:"WPI_UtilitiesGetTreeIOName.vi"("NewVal"=w292, "TreeControl in"=w294) -> ("I/O Name"=w295:string)  [unwired: 9 in]
        n153 = case shown="\"Analog Out\", \"Motor\", \"PWM\"" w295 {
          selector: w295 -> [_ w302 _ w324 w333 _]
          tunnel: w292 -> [_ _ w321 w323 _ w340]
          tunnel: w291 -> [_ _ _ _ _ w339]
          frame Default {
            w297 = FALSE ("Visible")
            w296 = FALSE ("Visible")
            n154 = property on="Motor" class="Clust (strict)"("Visible"=w296) -> ()  [unwired: 2 in, 2 out]
            n155 = property on="Test Ring" class="Ring (strict)"("Visible"=w296) -> ()  [unwired: 2 in, 2 out]
            n156 = property on="Rev/Fwd" class="Clust (strict)"("Visible"=w297) -> ()  [unwired: 2 in, 2 out]
            n157 = property on="On/Off" class="Bool (strict)"("Visible"=w297) -> ()  [unwired: 2 in, 2 out]
            n158 = property on="Test Slider" class="Slide (strict)"("Visible"=w297) -> ()  [unwired: 2 in, 2 out]
          }
          frame "Analog Out", "Motor", "PWM" {
            w303 = FALSE ("Visible")
            n159 = case shown="\"Analog Out\"" w302 {
              tunnel: [1.0 ("Value") -1.0 ("Value") 0.0 ("Value")] -> w301
              tunnel: [255.0 ("Value") 1.0 ("Value") 5.0 ("Value")] -> w300
              tunnel: [128.0 ("Value") 0.0 ("Value") 0.0 ("Value")] -> w299
              tunnel: [64.0 ("Value") 0.5 ("Value") 1.0 ("Value")] -> w298
              frame "PWM" {
              }
              frame "Motor", Default {
              }
              frame "Analog Out" {
              }
            }
            n160 = property on="Motor" class="Clust (strict)"("Visible"=TRUE) -> ()  [unwired: 2 in, 2 out]
            n161 = property on="Value" class="Slide (strict)"("Value"=w299, "Scale.Minimum"=w301, "Scale.Maximum"=w300, "Scale.Increment"=w298) -> ()  [unwired: 2 in, 2 out]
            n162 = property on="On/Off" class="Bool (strict)"("Visible"=w303) -> ()  [unwired: 2 in, 2 out]
            n163 = property on="Test Slider" class="Slide (strict)"("Visible"=w303) -> ()  [unwired: 2 in, 2 out]
            n164 = property on="Test Ring" class="Ring (strict)"("Visible"=w303) -> ()  [unwired: 2 in, 2 out]
            n165 = property on="Rev/Fwd" class="Clust (strict)"("Visible"=w303) -> ()  [unwired: 2 in, 2 out]
          }
          frame "Servo" {
            w319 = FALSE ("Visible")
            n166 = call <vilib>:"NT Read Number.vi"("Name"=w321) -> ("Numeric"=w320:dbl)  [unwired: 9 in, 1 out]
            n167 = property on="Test Slider" class="Slide (strict)"("Visible"=TRUE, "Scale.Maximum"=170.0 ("Scale.Range:Maximum")) -> ()  [unwired: 2 in, 2 out]
            n168 = local write "Test Slider"(w320) -> ()
            n169 = property on="Motor" class="Clust (strict)"("Visible"=w319) -> ()  [unwired: 2 in, 2 out]
            n170 = property on="Rev/Fwd" class="Clust (strict)"("Visible"=w319) -> ()  [unwired: 2 in, 2 out]
            n171 = property on="On/Off" class="Bool (strict)"("Visible"=w319) -> ()  [unwired: 2 in, 2 out]
            n172 = property on="Test Ring" class="Ring (strict)"("Visible"=w319) -> ()  [unwired: 2 in, 2 out]
          }
          frame "Relay", "Solenoid" {
            w322 = FALSE ("Visible")
            n173 = property on="Motor" class="Clust (strict)"("Visible"=w322) -> ()  [unwired: 2 in, 2 out]
            n174 = property on="Test Slider" class="Slide (strict)"("Visible"=w322) -> ()  [unwired: 2 in, 2 out]
            n175 = Search and Replace String(input string=w323, search string="/Value  **", replace string="/Direction") -> (result string=w329:string)  [unwired: 5 in, 3 out]
            n176 = property on="Test Ring" class="Ring (strict)"("Visible"=w322) -> ()  [unwired: 2 in, 2 out]
            n177 = call <vilib>:"NT Read String.vi"("Name"=w329) -> ("String"=w327:string)  [unwired: 9 in, 1 out]
            n178 = Equal?(x="Both directions", y=w327) -> (x = y?=w325:bool)
            n179 = Not(x=w325) -> (.not. x?=w326:bool)
            n180 = property on="Rev/Fwd" class="Clust (strict)"("Visible"=w325) -> ()  [unwired: 2 in, 2 out]
            n181 = property on="On/Off" class="Bool (strict)"("Visible"=w326, "Caption.Text"=w324) -> ()  [unwired: 2 in, 2 out]
          }
          frame "Compressor", "Digital Out" {
            w332 = FALSE ("Visible")
            # "Get direction and finish"
            n182 = property on="Motor" class="Clust (strict)"("Visible"=w332) -> ()  [unwired: 2 in, 2 out]
            n183 = property on="Test Slider" class="Slide (strict)"("Visible"=w332) -> ()  [unwired: 2 in, 2 out]
            n184 = property on="Test Ring" class="Ring (strict)"("Visible"=w332) -> ()  [unwired: 2 in, 2 out]
            n185 = property on="On/Off" class="Bool (strict)"("Visible"=TRUE, "Caption.Text"=w333) -> ()  [unwired: 2 in, 2 out]
            n186 = property on="Rev/Fwd" class="Clust (strict)"("Visible"=FALSE) -> ()  [unwired: 2 in, 2 out]
          }
          frame "Camera" {
            n187 = call <vilib>:"Get Last Path Segment.vi"("String in"=w340) -> ("String out"=w341:string)  [unwired: 10 in]
            n188 = property on="On/Off" class="Bool (strict)"("Visible"=FALSE) -> ()  [unwired: 2 in, 2 out]
            n189 = property on="Motor" class="Clust (strict)"("Visible"=FALSE) -> ()  [unwired: 2 in, 2 out]
            n190 = property on="Rev/Fwd" class="Clust (strict)"("Visible"=FALSE) -> ()  [unwired: 2 in, 2 out]
            n191 = case shown="\"White Balance  **\"" w341 {
              tunnel: w340 -> [w347 w356 w365 w374 w383 _ w389]
              tunnel: w339 -> [w345 w353 w362 w371 w380 _ _]
              frame "Size  **" {
                n192 = Index Array(array=w345) -> (element=w344:cluster{string[]})  [unwired: 1 in]
                n193 = call <vilib>:"NT Read String.vi"("Name"=w347) -> ("String"=w346:string)  [unwired: 9 in, 1 out]
                n194 = Unbundle(w344) -> (w342:string[])
                n195 = Match First String(2:w342, 3:w346) -> (0:w343:i32)  [unwired: 1 out]
                n196 = property on="Test Ring" class="Ring (strict)"("Value"=w343, "Strings []"=w342) -> ()  [unwired: 2 in, 2 out]
                n197 = property on="Test Ring" class="Ring (strict)"("Visible"=TRUE) -> ()  [unwired: 2 in, 2 out]
                n198 = property on="Test Slider" class="Slide (strict)"("Visible"=FALSE) -> ()  [unwired: 2 in, 2 out]
              }
              frame "White Balance  **" {
                n199 = Index Array(array=w353, index=1) -> (element=w354:cluster{string[]})
                n200 = call <vilib>:"NT Read String.vi"("Name"=w356) -> ("String"=w355:string)  [unwired: 9 in, 1 out]
                n201 = Unbundle(w354) -> (w351:string[])
                n202 = Match First String(2:w351, 3:w355) -> (0:w350:i32)  [unwired: 1 out]
                n203 = property on="Test Ring" class="Ring (strict)"("Value"=w350, "Strings []"=w351) -> ()  [unwired: 2 in, 2 out]
                n204 = property on="Test Ring" class="Ring (strict)"("Visible"=TRUE) -> ()  [unwired: 2 in, 2 out]
                n205 = property on="Test Slider" class="Slide (strict)"("Visible"=FALSE) -> ()  [unwired: 2 in, 2 out]
              }
              frame "Exposure  **" {
                n206 = Index Array(array=w362, index=2) -> (element=w363:cluster{string[]})
                n207 = call <vilib>:"NT Read String.vi"("Name"=w365) -> ("String"=w364:string)  [unwired: 9 in, 1 out]
                n208 = Unbundle(w363) -> (w359:string[])
                n209 = Match First String(2:w359, 3:w364) -> (0:w360:i32)  [unwired: 1 out]
                n210 = property on="Test Ring" class="Ring (strict)"("Value"=w360, "Strings []"=w359) -> ()  [unwired: 2 in, 2 out]
                n211 = property on="Test Ring" class="Ring (strict)"("Visible"=TRUE) -> ()  [unwired: 2 in, 2 out]
                n212 = property on="Test Slider" class="Slide (strict)"("Visible"=FALSE) -> ()  [unwired: 2 in, 2 out]
              }
              frame "Exposure Priority  **" {
                n213 = Index Array(array=w371, index=3) -> (element=w372:cluster{string[]})
                n214 = call <vilib>:"NT Read String.vi"("Name"=w374) -> ("String"=w373:string)  [unwired: 9 in, 1 out]
                n215 = Unbundle(w372) -> (w368:string[])
                n216 = Match First String(2:w368, 3:w373) -> (0:w369:i32)  [unwired: 1 out]
                n217 = property on="Test Ring" class="Ring (strict)"("Value"=w369, "Strings []"=w368) -> ()  [unwired: 2 in, 2 out]
                n218 = property on="Test Ring" class="Ring (strict)"("Visible"=TRUE) -> ()  [unwired: 2 in, 2 out]
                n219 = property on="Test Slider" class="Slide (strict)"("Visible"=FALSE) -> ()  [unwired: 2 in, 2 out]
              }
              frame "Color Enable  **" {
                n220 = Index Array(array=w380, index=4) -> (element=w381:cluster{string[]})
                n221 = call <vilib>:"NT Read String.vi"("Name"=w383) -> ("String"=w382:string)  [unwired: 9 in, 1 out]
                n222 = Unbundle(w381) -> (w377:string[])
                n223 = Match First String(2:w377, 3:w382) -> (0:w378:i32)  [unwired: 1 out]
                n224 = property on="Test Ring" class="Ring (strict)"("Value"=w378, "Strings []"=w377) -> ()  [unwired: 2 in, 2 out]
                n225 = property on="Test Ring" class="Ring (strict)"("Visible"=TRUE) -> ()  [unwired: 2 in, 2 out]
                n226 = property on="Test Slider" class="Slide (strict)"("Visible"=FALSE) -> ()  [unwired: 2 in, 2 out]
              }
              frame Default {
                n227 = property on="Test Ring" class="Ring (strict)"("Visible"=FALSE) -> ()  [unwired: 2 in, 2 out]
                n228 = property on="Test Slider" class="Slide (strict)"("Visible"=FALSE) -> ()  [unwired: 2 in, 2 out]
              }
              frame "Brightness  **", "Color Level  **", "Compression  **", "FPS  **", "Sharpness  **" {
                n229 = call <vilib>:"NT Read Number.vi"("Name"=w389) -> ("Numeric"=w388:dbl)  [unwired: 9 in, 1 out]
                n230 = local write "Test Slider"(w388) -> ()
                n231 = property on="Test Slider" class="Slide (strict)"("Visible"=TRUE, "Scale.Maximum"=100.0 ("Scale.Range:Maximum")) -> ()  [unwired: 2 in, 2 out]
                n232 = property on="Test Ring" class="Ring (strict)"("Visible"=FALSE) -> ()  [unwired: 2 in, 2 out]
              }
            }
          }
        }
        n233 = property on="Progress" class="Clust (strict)"("Visible"=FALSE) -> ()  [unwired: 2 in, 2 out]
      }
      event "Test Name": Mouse Enter {
        # "Populate the ring with the list of tests"
        n234 = event-data() -> ()  [unwired: 1 in, 1 out]
        n235 = call <vilib>:"NT Read String Array.vi"("Name"="/TestMode/TestList") -> ("String Array"=w398:string[])  [unwired: 9 in, 1 out]
        n236 = Build Array (concatenate)("Select the test to run...", w398) -> (w397:string[])
        n237 = property on="Test Name" class="Ring (strict)"("Strings []"=w397) -> ()  [unwired: 2 in, 2 out]
      }
      event "Test Name": Value Change {
        w401 = FALSE ("Visible")
        # "Tell the robot the test name to run"
        n238 = event-data() -> ("NewVal"=w405:u16)  [unwired: 1 in]
        n239 = property on="Test Name" class="Ring (strict)"() -> ("Strings []"=w406:string[])  [unwired: 2 in, 2 out]
        n240 = local write "Progress"(T5 {"Test Progress"=0, "Test Progress Text"=""} ("Progress")) -> ()
        n241 = Index Array(array=w406, index=w405) -> (element=w404:string)
        n242 = call <vilib>:"NT Write String.vi"("String"=w404, "Name"="/TestMode/TestName") -> ()  [unwired: 9 in, 1 out]
        n243 = property on="Progress" class="Clust (strict)"("Visible"=TRUE) -> ()  [unwired: 2 in, 2 out]
        n244 = property on="Motor" class="Clust (strict)"("Visible"=w401) -> ()  [unwired: 2 in, 2 out]
        n245 = property on="Test Slider" class="Slide (strict)"("Visible"=w401) -> ()  [unwired: 2 in, 2 out]
        n246 = property on="On/Off" class="Bool (strict)"("Visible"=w401) -> ()  [unwired: 2 in, 2 out]
        n247 = property on="Rev/Fwd" class="Clust (strict)"("Visible"=w401) -> ()  [unwired: 2 in, 2 out]
        n248 = property on="Test Ring" class="Ring (strict)"("Visible"=w401) -> ()  [unwired: 2 in, 2 out]
      }
      event "Command Selection": Value Change {
        # "Get the params and show in table"
        n249 = event-data() -> ("NewVal"=w411:i32)  [unwired: 1 in]
        n250 = property on="Command Selection" class="MCListbox (strict)"() -> ("ItemNames"=w409:string[][])  [unwired: 2 in, 2 out]
        n251 = call <vilib>:"WPI_DashboardUpdate Command Params.vi"("NewVal"=w411, "Commands"=w409, "Param Tbl"=w410) -> ()  [unwired: 8 in, 1 out]
      }
      event "Execute Command": Value Change {
        # "Started one, Unique ID holds\nresponse"
        n252 = event-data() -> ()  [unwired: 1 in, 1 out]
        n253 = property on="Command Selection" class="MCListbox (strict)"() -> ("ItemNames"=w423:string[][])  [unwired: 2 in, 2 out]
        n254 = Index Array(array=w423, index (row)="Command Selection", index (col)=0) -> (element=w421:string)
        n255 = call <vilib>:"Invoke Commands.vi"("Command Params"="Command Params", "Function Name"=w421) -> ("Params"=w417:u8, "Started"=w416:bool)  [unwired: 7 in, 1 out]
        n256 = Array Subset(array="Command Params", length (row)=w417) -> (w418:string[][])  [unwired: 3 in]
        n257 = Select(t="Executing" ("Cmd Status"), s=w416, f="" ("Cmd Status")) -> (s? t:f=→"Cmd Status":string)
      }
      event "Command Selection": Double Click {
        n258 = event-data() -> ("Row"=w433:i32)  [unwired: 1 in]
        n259 = property on="Command Selection" class="MCListbox (strict)"() -> ("ItemNames"=w436:string[][])  [unwired: 2 in, 2 out]
        n260 = local read "Command Params"() -> (w431:string[][])
        n261 = Index Array(array=w436, index (row)=w433, index (col)=0) -> (element=w434:string)
        n262 = call <vilib>:"Invoke Commands.vi"("Command Params"=w431, "Function Name"=w434) -> ("Params"=w430:u8, "Started"=w425:bool)  [unwired: 7 in, 1 out]
        n263 = Array Subset(array=w431, length (row)=w430) -> (w429:string[][])  [unwired: 3 in]
        n264 = Select(t="Executing" ("Cmd Status"), s=w425, f="" ("Cmd Status")) -> (s? t:f=w426:string)
        n265 = local write "Cmd Status"(w426) -> ()
      }
      event "CheckList": Double Click {
        # "Shift clears all"
        # "Update symbols on the listbox"
        n266 = event-data() -> ("PlatMods.Shift"=w439:bool, "Row"=w441:i32)  [unwired: 1 in]
        n267 = case shown="True" w439 {
          tunnel: w441 -> [w445 _]
          tunnel: 1 -> [w444 _]
          frame False {
            n268 = property on="CheckList" class="LstBox (strict)"() -> ("Item Symbols"=w443:i32[])  [unwired: 2 in, 2 out]
            n269 = Replace Array Subset(array=w443, new element=w444, index=w445) -> (w442:i32[])
            n270 = property on="CheckList" class="LstBox (strict)"("Item Symbols"=w442) -> ()  [unwired: 2 in, 2 out]
          }
          frame True {
            w446 = 0 ("Top Row")
            n271 = property on="CheckList" class="LstBox (strict)"() -> ("Number of Rows"=w448:u32)  [unwired: 2 in, 2 out]
            n272 = Initialize Array(0, w448) -> (w447:i32[])
            n273 = property on="CheckList" class="LstBox (strict)"("Top Row"=w446, "Value"=w446, "Item Symbols"=w447) -> ()  [unwired: 2 in, 2 out]
          }
        }
      }
      event "CheckList": Key Down {
        # "Update symbols on the listbox\nLeft and right keys check and uncheck"
        n274 = event-data() -> ("VKey"=w453:T16)  [unwired: 1 in]
        n275 = case shown="\"Left\", \"Right\"" w453 {
          selector: w453 -> [w458 _]
          tunnel: eventvkey."Left" ("VKey") -> [w456 _]
          frame "Left", "Right" {
            n276 = Equal?(x=w456, y=w458) -> (x = y?=w457:bool)
            n277 = Select(t=0, s=w457, f=1) -> (s? t:f=w459:i32)
            n278 = property on="CheckList" class="LstBox (strict)"() -> ("Item Symbols"=w462:i32[])  [unwired: 2 in, 2 out]
            n279 = Replace Array Subset(array=w462, new element=w459, index="CheckList") -> (w461:i32[])
            n280 = property on="CheckList" class="LstBox (strict)"("Item Symbols"=w461) -> ()  [unwired: 2 in, 2 out]
          }
          frame Default {
          }
        }
      }
      event "DB Camera Config": Value Change {
        # "Show or hide the cluster of controls, store in ini file"
        n281 = event-data() -> ("NewVal"=w467:bool)  [unwired: 1 in]
        n282 = case shown="False" w467 {
          tunnel: w466 -> [w476 _]
          tunnel: [w469 w487] -> w465
          tunnel: w464 -> [w468 w487]
          frame False {
            w483 = "Camera"
            w486 = FALSE ("Visible")
            n283 = local read "Camera Settings"() -> (w475:T2)
            n284 = Index Array(array=w476) -> (element=w479:cluster{string[]})  [unwired: 1 in]
            n285 = Unbundle(w475) -> ("Frame Rate"=w474:i32, "Compression"=w473:i32, "Size"=w477:u16)
            n286 = Unbundle(w479) -> (w478:string[])
            n287 = Index Array(array=w478, index=w477) -> (element=w472:string)
            n288 = call-poly <vilib>:"Write Key.vi"("section"=w483, "value"=w472, "key"="Size", "refnum"=w468) -> ("refnum out"=w485:T14)  [unwired: 2 in, 5 out]
            n289 = call-poly <vilib>:"Write Key.vi"("section"=w483, "value"=w474, "key"="FrameRate", "refnum"=w485) -> ("refnum out"=w484:T14)  [unwired: 1 in, 6 out]
            n290 = property on="Camera Settings" class="Clust (strict)"("Visible"=w486) -> ()  [unwired: 2 in, 2 out]
            n291 = local write "DB Camera Config"(w486) -> ()
            n292 = call-poly <vilib>:"Write Key.vi"("section"=w483, "value"=w473, "key"="Compression", "refnum"=w484) -> ("refnum out"=w470:T14)  [unwired: 1 in, 6 out]
            n293 = call <vilib>:"Close Config Data.vi"("refnum"=w470) -> ("file path"=w471:path)  [unwired: 2 in, 8 out]
            n294 = call <vilib>:"Open Config Data.vi"("configuration file path"=w471) -> ("refnum"=w469:T14)  [unwired: 8 in, 2 out]
          }
          frame True {
            n295 = property on="Camera Settings" class="Clust (strict)"("Visible"=TRUE) -> ()  [unwired: 2 in, 2 out]
          }
        }
      }
      event "Camera Settings": Value Change {
        # "Update summary string when any elements of DB camera change"
        n296 = event-data() -> ("NewVal"=w501:T2)  [unwired: 1 in]
        n297 = Index Array(array=w497) -> (element=w496:cluster{string[]})  [unwired: 1 in]
        n298 = Unbundle(w501) -> ("Frame Rate"=w492:i32, "Compression"=w491:i32, "Size"=w494:u16)
        n299 = Unbundle(w496) -> (w495:string[])
        n300 = Index Array(array=w495, index=w494) -> (element=w493:string)
        n301 = Format Into String(format string="%s   %dfps   %d%%", w493, w492, w491) -> (resulting string=w498:string)  [unwired: 2 in, 1 out]
        n302 = Build Array(w498) -> (w499:string[])
        n303 = property on="DB Camera Config" class="Bool (strict)"("Strings [4]"=w499) -> ()  [unwired: 2 in, 2 out]
      }
      event "Motor.Enable": Value Change {
        # "When the test mode otor enable helper is set, update that\ntree row item's value"
        n304 = event-data() -> ("NewVal"=w508:bool)  [unwired: 1 in]
        n305 = Unbundle("Motor") -> ("Value"=w507:dbl)  [unwired: 1 out]
        n306 = Select(t=w507, s=w508, f=0.0) -> (s? t:f=w505:dbl)
        n307 = call <vilib>:"NT Write Number.vi"("Numeric"=w505, "Name"=w504) -> ()  [unwired: 9 in, 1 out]
      }
      event "Test Slider": Value Change {
        # "When the test mode slider helper is set, update that\ntree row item's value"
        n308 = event-data() -> ("NewVal"=w512:dbl)  [unwired: 1 in]
        n309 = call <vilib>:"NT Write Number.vi"("Numeric"=w512, "Name"=w513) -> ()  [unwired: 9 in, 1 out]
      }
      event "On/Off": Value Change {
        # "When the test mode on/off helper value is set, update that\ntree row item's value"
        n310 = event-data() -> ("NewVal"=w518:bool)  [unwired: 1 in]
        n311 = Boolean To (0,1)(Boolean=w518) -> (0, 1=w517:i16)
        n312 = call <vilib>:"NT Write Number.vi"("Numeric"=w517, "Name"=w516) -> ()  [unwired: 9 in, 1 out]
      }
      event "Rev/Fwd": Value Change {
        # "When the test mode helper value for relays is set, update that\ntree row item's value"
        n313 = event-data() -> ("NewVal.Forward"=w527:bool, "NewVal.Reverse"=w526:bool)  [unwired: 1 in]
        n314 = Boolean To (0,1)(Boolean=w527) -> (0, 1=w523:i16)
        n315 = Boolean To (0,1)(Boolean=w526) -> (0, 1=w525:i16)
        n316 = Negate(x=w525) -> (-x=w524:i16)
        n317 = Add(x=w523, y=w524) -> (x+y=w522:i16)
        n318 = call <vilib>:"NT Write Number.vi"("Numeric"=w522, "Name"=w521) -> ()  [unwired: 9 in, 1 out]
      }
      event "Test Ring": Value Change {
        # "When a test mode helper value is selected from the ring,\nset the tree item's variable to the string value"
        n319 = event-data() -> ("NewVal"=w532:u16)  [unwired: 1 in]
        n320 = property on="Test Ring" class="Ring (strict)"() -> ("Strings []"=w533:string[])  [unwired: 2 in, 2 out]
        n321 = Index Array(array=w533, index=w532) -> (element=w531:string)
        n322 = call <vilib>:"NT Write String.vi"("String"=w531, "Name"=w530) -> ()  [unwired: 9 in, 1 out]
      }
      event "Rec Mode": Value Change {
        # "Update globals for recording mode and path to read log from.\nClear when logging and let NetworkTables set path for vision to\nuse."
        n323 = event-data() -> ("NewVal"=w545:enum32{"Stop", "Record", "Playback"})  [unwired: 1 in]
        n324 = global write "WPI_DashboardLogging Global.vi" "Logging Filename"(path "") -> ()
        n325 = global write "WPI_DashboardLogging Global.vi" "Recording"(w545) -> ()
        n326 = case shown="\"Playback\"" w545 {
          tunnel: w544 -> [_ w547 w556]
          tunnel: [_ _ w555] -> w541
          tunnel: [_ _ w554] -> _
          tunnel: w539 -> [_ _ w552]
          tunnel: cluster{i32, i32} {-250, 170} -> [_ _ w551]
          tunnel: [_ _ T17 {"Image Size"=TRUE, "Image Type"=TRUE, "Pixel Value"=TRUE, "ROI Information"=TRUE, "Zoom Factor"=FALSE} ("Image Information Shown:All Elements")] -> w537
          tunnel: [_ _ TRUE ("Zoom Factor")] -> w536
          tunnel: w535 -> [_ _ w548]
          frame Default {
          }
          frame "Stop", "Record" {
            # "Place Window too"
            n327 = invoke class="VI" method="FP.Close"(reference=w547) -> (reference out=w546:refnum<vi>)  [unwired: 2 in, 2 out]
            n328 = invoke class="VI" method="Abort VI"(reference=w546) -> ()  [unwired: 2 in, 3 out]
          }
          frame "Playback" {
            n329 = call "Open Playback Panel.vi"("Offset"=w551, "DB VI Ref"=w552, "Playback in"=w556) -> ("Playback out"=w553:refnum<vi>)  [unwired: 8 in]
            n330 = register-events(w553, w548) -> (reference out=w555:refnum<event-registration>, error out=w554:errorcluster)  [unwired: 2 in]
          }
        }
        n331 = property on="Camera Image" class="ImageControl"("Image Information Shown"=w537, "Image Information Visible"=w536) -> ()  [unwired: 2 in, 2 out]
        n332 = call <vilib>:"WPI_DashboardNT Log FieldName Cache.vi"("Operation"=enum16{"Lookup/Add", "Index", "Clear"}."Clear") -> ()  [unwired: 8 in, 3 out]
      }
      event Panel Close {
        w558 = enum32{"Stop", "Record", "Playback"}."Stop" ("Rec Mode")
        # "Playback window has been closed, abort"
        n333 = event-data() -> ()  [unwired: 1 in, 4 out]
        n334 = local write "Rec Mode"(w558) -> ()
        n335 = global write "WPI_DashboardLogging Global.vi" "Recording"(w558) -> ()
      }
      event Panel Close {
        # "Abort playback window and ourself"
        n336 = event-data() -> ()  [unwired: 1 in, 4 out]
        n337 = invoke class="VI" method="FP.Close"(reference=w564) -> (reference out=w563:refnum<vi>)  [unwired: 2 in, 2 out]
        n338 = invoke class="VI" method="Abort VI"(reference=w563) -> (error out=w562:errorcluster)  [unwired: 2 in, 2 out]
        n339 = invoke class="VI" method="Abort VI"(error in=w562) -> ()  [unwired: 2 in, 3 out]
      }
      event User Event {
        n340 = event-data() -> ("IDs"=w572:cluster{"RPC field ID":u16, "Unique ID":u16}, "String"=w571:string)  [unwired: 1 in]
        n341 = Bundle("IDs"=w572, "String"=w571) -> (w570:T6)  [unwired: 1 in]
        n342 = call <vilib>:"Retrieve RPC Response.vi"("RPC Response"=w570) -> ("Output"=w567:string[][])  [unwired: 10 in]
        n343 = Build Array (concatenate)(w565, w567) -> (w566:string[][])
        n344 = local write "Command Params"(w566) -> ()
        n345 = local write "Cmd Status"("" ("Cmd Status")) -> ()
      }
      event "Vision": Value Change {
        # "Enable/Disable Compression slider.\nHW USB is hard-coded into the camera"
        n346 = event-data() -> ("NewVal"=w579:u16)  [unwired: 1 in]
        n347 = Equal?(x=w579, y=u32 2 ("milliseconds to wait")) -> (x = y?=w577:bool)
        n348 = Select(t=T18."Disabled and Grayed Out" ("Disabled"), s=w577, f=T18."Enabled" ("Disabled")) -> (s? t:f=w574:T18)
        n349 = property on="Compression" class="Slide (strict)"("DisabledEnum"=w574) -> ()  [unwired: 2 in, 2 out]
      }
      event "Tree": Double Click {
        n350 = event-data() -> ("PlatMods"=w584:T21, "Tag"=w583:string)  [unwired: 1 in]
        n351 = Unbundle(w584) -> ("Shift"=w582:bool)  [unwired: 4 out]
        n352 = Not(x=w582) -> (.not. x?=w581:bool)
        n353 = call <vilib>:"NT Update Persistence.vi"("Persistence"=w581, "Name"=w583) -> ()  [unwired: 9 in, 1 out]
      }
    }
  }
  n354 = while {
    tunnel: w28 -> [w588]
    i -> [w591]
    stop <- FALSE stop-if-true
    n355 = Wait (ms)(milliseconds to wait=u32 100) -> ()  [unwired: 1 out]
    n356 = case shown="\"Playback\"" "Rec Mode" {
      tunnel: w591 -> [_ _ w606]
      tunnel: [u32 2829099 ("Base Color") u32 11141120 ("Target Color") w595] -> w587
      frame "Stop", Default {
        # "Reset the color, extra updates don't cost much"
      }
      frame "Record" {
      }
      frame "Playback" {
        # "Playback"
        n357 = Quotient & Remainder(x=w606, y=u32 50 ("milliseconds to wait")) -> (x-y*floor(x/y)=w602:u32)  [unwired: 1 out]
        n358 = Divide(x=w602, y=u32 50 ("milliseconds to wait")) -> (x/y=w599:dbl)
        n359 = Multiply(x=6.283185307179586, y=w599) -> (x*y=w604:dbl)
        n360 = Sine(x=w604) -> (sin(x)=w603:dbl)
        n361 = Absolute Value(x=w603) -> (abs(x)=w596:dbl)
        n362 = call "Interpolate RGB Color.vi"("Proportion"=w596, "Target Color"=u32 30976, "Base Color"=u32 2829099) -> ("Result Color"=w595:u32)  [unwired: 8 in]
      }
    }
    n363 = property class="Pane"(reference=w588, "PaneColor"=w587) -> ()  [unwired: 1 in, 2 out]
  }
  n364 = local write "Dashboard Tab"(T1."Test" ("Dashboard Tab")) -> ()
  n365 = property on="On/Off" class="Bool (strict)"("Visible"=w11) -> ()  [unwired: 2 in, 2 out]
  n366 = property on="Motor" class="Clust (strict)"("Visible"=w11) -> ()  [unwired: 2 in, 2 out]
  n367 = property on="Progress" class="Clust (strict)"("Visible"=w11) -> ()  [unwired: 2 in, 2 out]
  n368 = property on="Test Ring" class="Ring (strict)"("Visible"=w11) -> ()  [unwired: 2 in, 2 out]
  n369 = property on="Rev/Fwd" class="Clust (strict)"("Visible"=w11) -> ()  [unwired: 2 in, 2 out]
  n370 = property on="Camera Settings" class="Clust (strict)"("Visible"=w11) -> ()  [unwired: 2 in, 2 out]
  n371 = local write "DB Camera Config"(w11) -> ()
  n372 = local write "Command Params"(string[][] [] ("Command Params")) -> ()
  n373 = global write "WPI_DashboardLogging Global.vi" "Recording"(w22) -> ()
  n374 = local write "Rec Mode"(w22) -> ()
  n375 = while {
    tunnel: u16 1741 ("timeout ms (25000)") -> [w608]
    stop <- FALSE stop-if-true
    n376 = TCP Create Listener(10:w608) -> (0:w607:errorcluster, 3:w609:refnum<k5>)  [unwired: 4 in, 1 out]
    n377 = case shown="No Error" w607 {
      selector: w607 -> [w611 _]
      tunnel: w609 -> [w612 _]
      frame No Error {
        n378 = while {
          tunnel: w612 -> [w615]
          tunnel: w611 -> [w614]
          stop <- FALSE stop-if-true
          n379 = TCP Wait On Listener(8:w614, 11:w615) -> (0:w616:errorcluster, 4:w617:refnum<k5>)  [unwired: 2 in, 3 out]
          n380 = local write "TCP"(w617) -> ()
          n381 = case shown="No Error" w616 {
            frame No Error {
            }
            frame Error {
              n382 = Wait (ms)(milliseconds to wait=u32 1000) -> ()  [unwired: 1 out]
            }
          }
        }
      }
      frame Error {
        n383 = Wait (ms)(milliseconds to wait=u32 1000) -> ()  [unwired: 1 out]
      }
    }
  }
  n384 = local write "Command Selection"(u16 0 ("milliseconds to wait")) -> ()
